vi "Get T & H DBL.vi"(11 "String Input":string=" T = 21.10, H = 2.03") -> (2 "H DBL":dbl, 3 "T DBL":dbl)   [LabVIEW 2018]
panel:
  out "H String":string
  out "T String":string
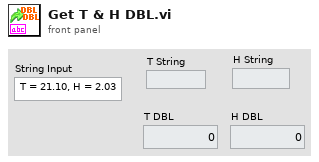
[diagram p1: front panel]
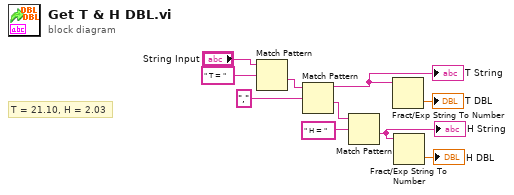
[diagram p0: block diagram]
diagram:
  # "T = 21.10, H = 2.03"
  n1 = Match Pattern(string="String Input", regular expression=" T = ") -> (after substring=w8:string)  [unwired: 1 in, 3 out]
  n2 = Match Pattern(string=w8, regular expression=",") -> (before substring=w4:string, after substring=w6:string)  [unwired: 1 in, 2 out]
  "T String" <- w4
  n3 = Match Pattern(string=w6, regular expression=" H = ") -> (after substring=w1:string)  [unwired: 1 in, 3 out]
  "H String" <- w1
  n4 = Fract/Exp String To Number(string=w4) -> (number=→"T DBL":dbl)  [unwired: 3 in, 1 out]
  n5 = Fract/Exp String To Number(string=w1) -> (number=→"H DBL":dbl)  [unwired: 3 in, 1 out]
